vi "ATEQwriteBit气密机一.vi"(8 "Write Address":u16 format="%x", 9 "baud rate":u32=57600 caption="波特率(9600)", 10 "VISA resource name":refnum<visa-resource-name>="COM3" caption="COM", 11 "从站地址":u8=2 format="%x") -> (3 "Write Status":bool)   [LabVIEW 2014]
uses:
  <vilib>/Instr/_visa.llb/VISA Configure Serial Port (Instr).vi
panel:
  out "ReturnWrite":string
  out "WriteSend":string
  out "Write Return Value":string
  out "Send Write Date":string
  out "Write Data":u16=65280 format="%x"
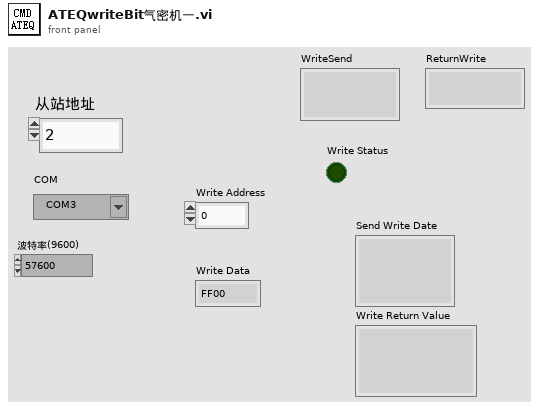
[diagram p1: front panel]
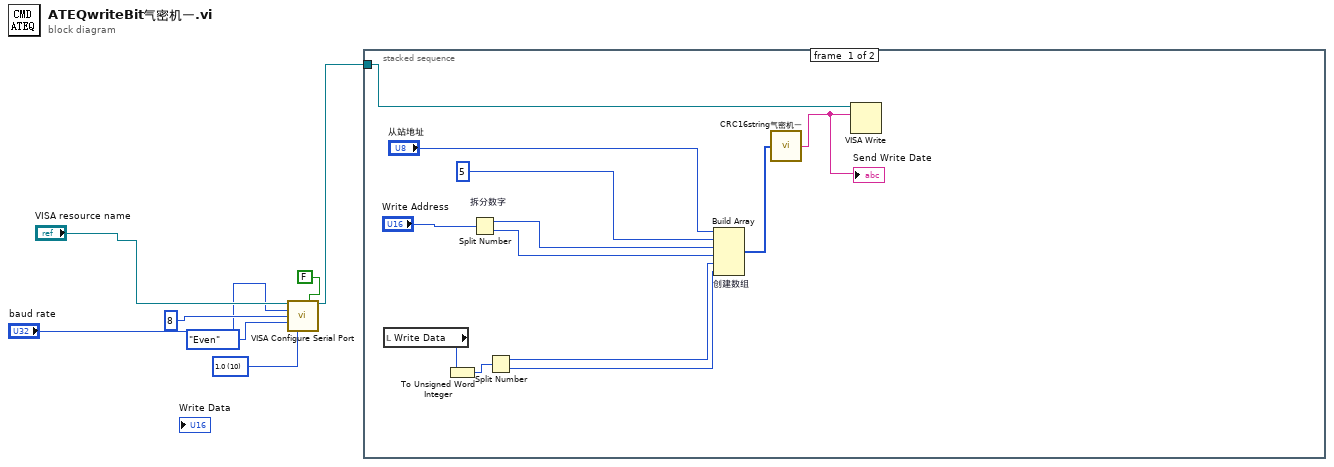
[diagram p0: block diagram]
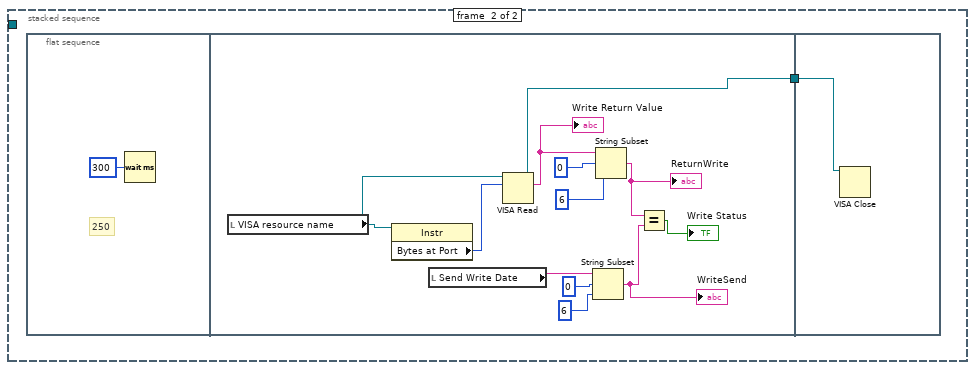
[diagram p2: hidden frame]
diagram:
  w7 = u16 10 items=["1.0"=10, "1.5"=15, "2.0"=20] ("stop bits (10: 1 bit)")
  n1 = call-poly "VISA Configure Serial Port"("VISA resource name"="VISA resource name", "Enable Termination\nChar (T)"=FALSE ("Enable Termination\nChar (T)"), "baud rate (9600)"="baud rate", "data bits (8)"=u16 8, "parity (0:none)"=enum16{"None", "Odd", "Even", "Mark", "Space"}."Even", "stop bits (10: 1 bit)"=w7) -> ("VISA resource name out"=w3:refnum<visa-resource-name>)  [unwired: 8 in, 1 out]
  n2 = stacked-sequence {
    tunnel: w3 -> [w14 _]
    frame #0 {
      n3 = local read "Write Data"() -> (w8:u16)
      n4 = To Unsigned Word Integer(number=w8) -> (unsigned 16bit integer=w19:u16)
      n5 = Split Number "拆分数字"(x="Write Address") -> (hi(x)=w17:u8, lo(x)=w16:u8)
      n6 = Split Number(x=w19) -> (hi(x)=w10:u8, lo(x)=w9:u8)
      n7 = Build Array "创建数组"("从站地址", u8 5, w17, w16, w10, w9) -> (w15:u8[])
      n8 = call "CRC16string气密机一.vi"("数组"=w15) -> ("要发送的数据"=w11:string)
      "Send Write Date" <- w11
      n9 = VISA Write(VISA resource name=w14, write buffer=w11) -> ()  [unwired: 1 in, 3 out]
    }
    frame #1 {
      n10 = flat-sequence {
        tunnel: [w22] -> w20
        tunnel: w20 -> [w34]
        frame #0 {
          # "250"
          n11 = Wait (ms)(milliseconds to wait=u32 300 ("等待时间（毫秒）")) -> ()  [unwired: 1 out]
        }
        frame #1 {
          n12 = local read "VISA resource name"() -> (w33:refnum<visa-resource-name>)
          n13 = property class="Instr"(reference=w33) -> ("Bytes at Port"=w32:u32)  [unwired: 1 in, 2 out]
          n14 = local read "Send Write Date"() -> (w30:string)
          n15 = VISA Read(VISA resource name=w33, byte count=w32) -> (VISA resource name out=w22:refnum<visa-resource-name>, read buffer=w29:string)  [unwired: 1 in, 2 out]
          "Write Return Value" <- w29
          n16 = String Subset(string=w30, offset (0)=0 ("偏移量(0)"), length (rest)=6 ("长度（剩余）")) -> (substring=w25:string)
          "WriteSend" <- w25
          n17 = String Subset(string=w29, offset (0)=0 ("偏移量(0)"), length (rest)=6 ("长度（剩余）")) -> (substring=w26:string)
          "ReturnWrite" <- w26
          n18 = Equal?(x=w26, y=w25) -> (x = y?=→"Write Status":bool)
        }
        frame #2 {
          n19 = VISA Close(VISA resource name=w34) -> ()  [unwired: 1 in, 1 out]
        }
      }
    }
  }
